vi "Get_Calbration_times.vi"(0 "File Path Control":path) -> (2 "CalNames":string[](array[string]), 3 "CalTimes":dbl[](array[numeric]) format="%<%Y-%m-%d  %H:%M:%S >T", 4 "CalPaths":path[](array[path]), 5 "CalDetails":T1(array[cluster]) {"Time Stamp Control" format="%<%Y-%m-%d  %H:%M:%S >T"})   [LabVIEW 2017]
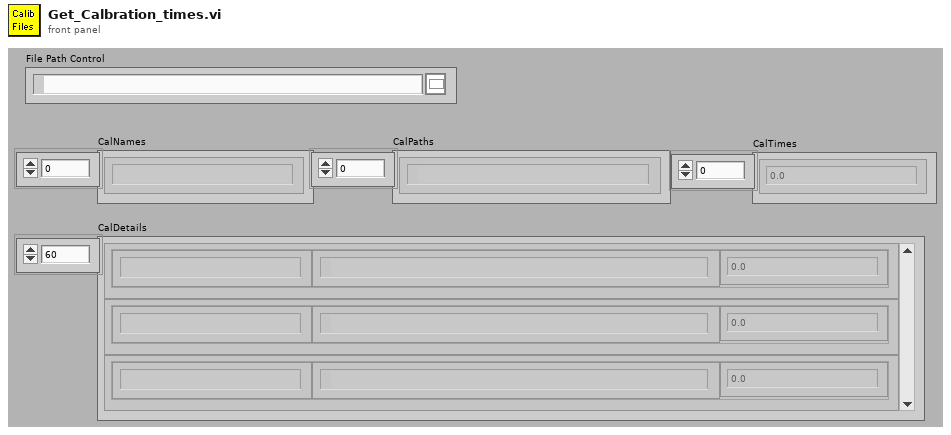
[diagram p1: front panel]
types:
  T1 = cluster{"String":string, "File Path Control":path, "Time Stamp Control":dbl}[]
  T2 = cluster{"CalFileName":string, "CalFilePath":path, "Timestamp":dbl}
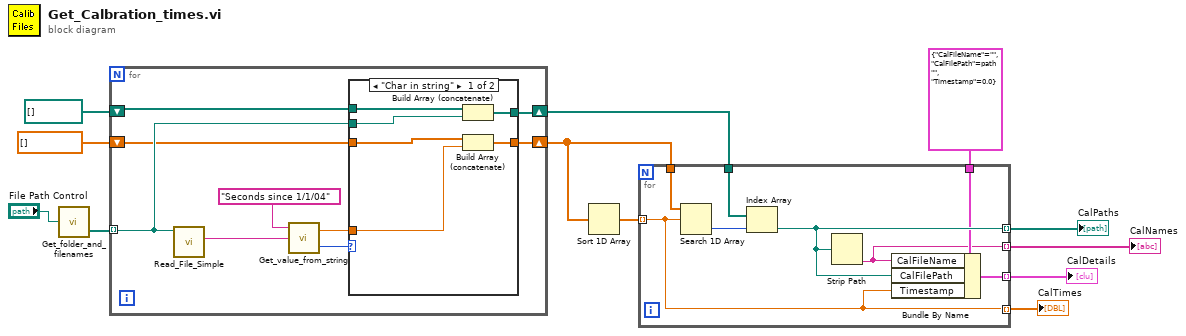
[diagram p0: block diagram]
diagram:
  n1 = call "Get_folder_and_filenames.vi"("file path (dialog if empty)"="File Path Control") -> ("Files"=w11:path[])  [unwired: 1 out]
  n2 = for {
    shift-right: [w17] -> w8
    shift-left: path[] [] -> [w19]
    shift-right: [w16] -> w7
    shift-left: dbl[] [] -> [w15]
    tunnel: w11 -> [w18] mode=indexing
    n3 = call "Read_File_Simple.vi"("Filename"=w18) -> ("string"=w13:string)  [unwired: 4 in, 5 out]
    n4 = call "Get_value_from_string.vi"("Input string"=w13, "Variable name"="Seconds since 1/1/04") -> ("Status"=w20:enum16{"Char in string", "Char not in string"}, "Value"=w14:dbl)  [unwired: 1 in]
    n5 = case shown="\"Char in string\"" w20 {
      tunnel: w19 -> [w27 w29]
      tunnel: w18 -> [w26 _]
      tunnel: [w25 w29] -> w17
      tunnel: [w24 w28] -> w16
      tunnel: w15 -> [w23 w28]
      tunnel: w14 -> [w22 _]
      frame "Char in string" {
        n6 = Build Array (concatenate)(w27, w26) -> (w25:path[])
        n7 = Build Array (concatenate)(w23, w22) -> (w24:dbl[])
      }
      frame "Char not in string" {
      }
    }
  }
  n8 = Sort 1D Array(array=w7) -> (sorted array=w12:dbl[])
  n9 = for {
    tunnel: w7 -> [w37]
    tunnel: w12 -> [w30] mode=indexing
    tunnel: w8 -> [w36]
    tunnel: [w34] -> w3 mode=indexing
    tunnel: T2 {"CalFileName"="", "CalFilePath"=path "", "Timestamp"=0.0} -> [w33]
    tunnel: [w32] -> w5 mode=indexing
    tunnel: [w31] -> w2 mode=indexing
    tunnel: [w30] -> w1 mode=indexing
    n10 = Search 1D Array(1D array=w37, element=w30) -> (index of element=w35:i32)  [unwired: 1 in]
    n11 = Index Array(array=w36, index=w35) -> (element=w34:path)
    n12 = Strip Path(path=w34) -> (name=w31:string)  [unwired: 1 out]
    n13 = Bundle By Name(cluster=w33, "CalFileName"=w31, "CalFilePath"=w34, "Timestamp"=w30) -> (w32:T2)
  }
  "CalDetails" <- w5
  "CalNames" <- w2
  "CalPaths" <- w3
  "CalTimes" <- w1
